vi "科学计算器.vi"() -> ()   [LabVIEW 2014]
panel:
  in  "右":T1
  in  "左":bool
  in  "↓":T2
  in  "↑":bool
  out "结果":string
  out "表达式":string
  in  "OFF":bool
  in  "BACKPLACE":bool
  in  "C":bool
  in  "ln":bool
  in  "^":bool
  in  "tan":bool
  in  "cos":bool
  in  "sin":bool
  in  ")":bool
  in  "(":bool
  in  ".":bool
  in  "=":bool
  in  "0":bool
  in  "9":bool
  in  "8":bool
  in  "7":bool
  in  "6":bool
  in  "5":bool
  in  "4":bool
  in  "3":bool
  in  "2":bool
  in  "1":bool
  in  "÷":bool
  in  "×":bool
  in  "-":bool
  in  "+":bool
  out "数值 2":dbl
  out "数值":dbl
  out "字符串":string
  out "左字":string
  # "小小计算器（科学型）"
  # "ssz"
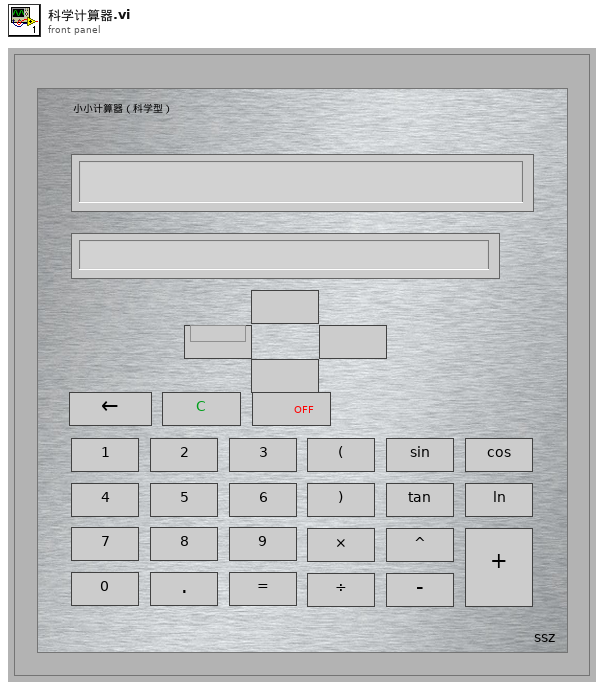
[diagram p1: front panel]
types:
  T1 = typedef "控件 3.ctl" = bool
  T2 = typedef "控件 2.ctl" = bool
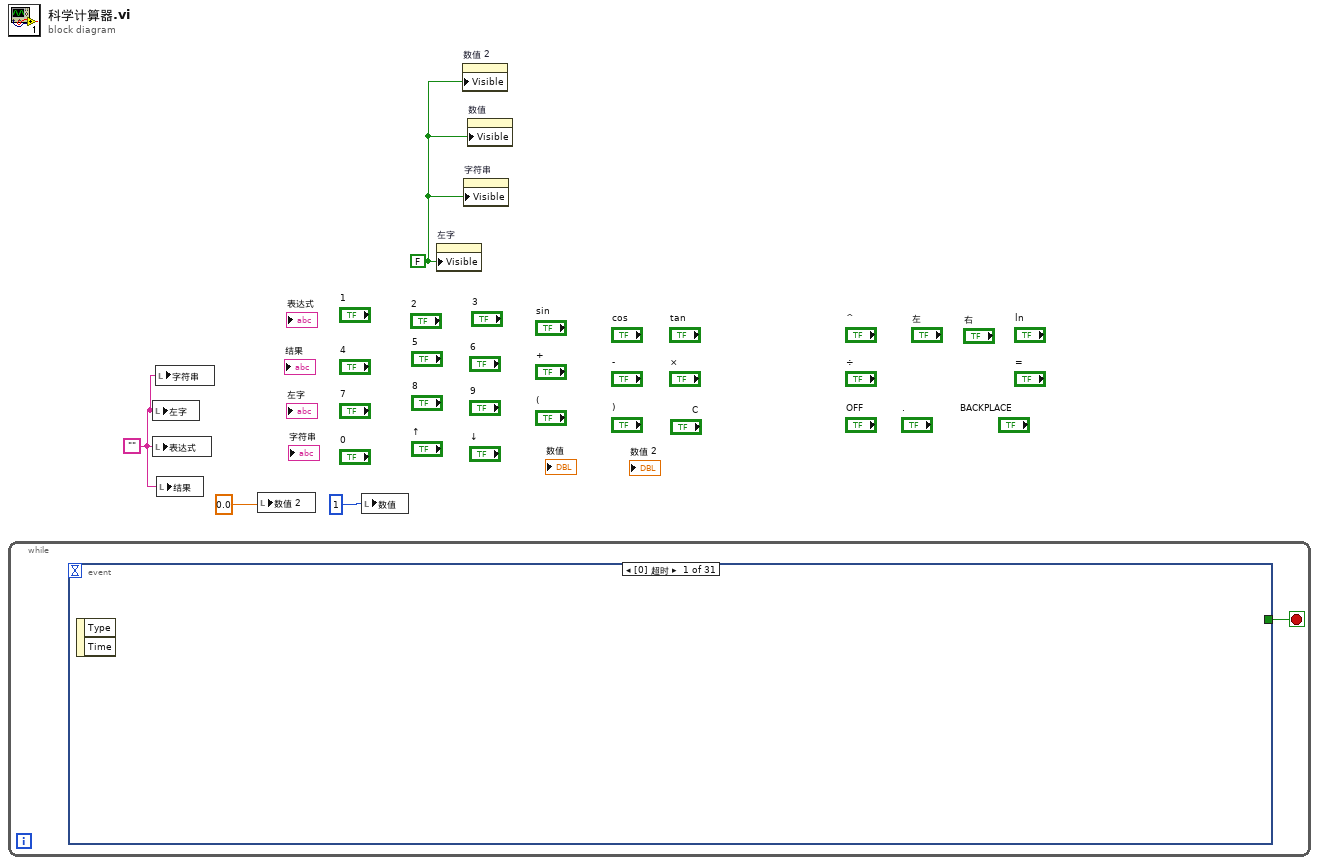
[diagram p0: block diagram]
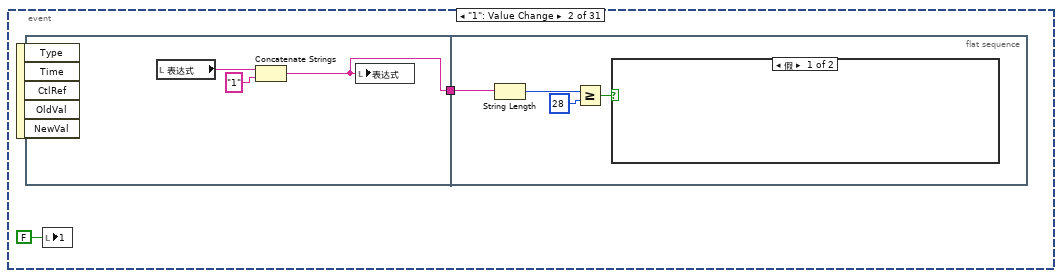
[diagram p2: hidden frame]
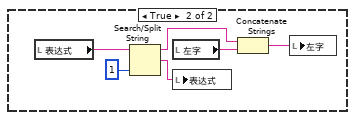
[diagram p3: hidden frame]
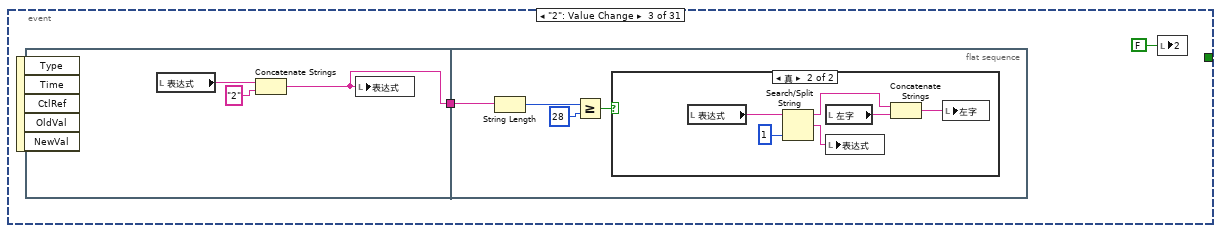
[diagram p4: hidden frame]
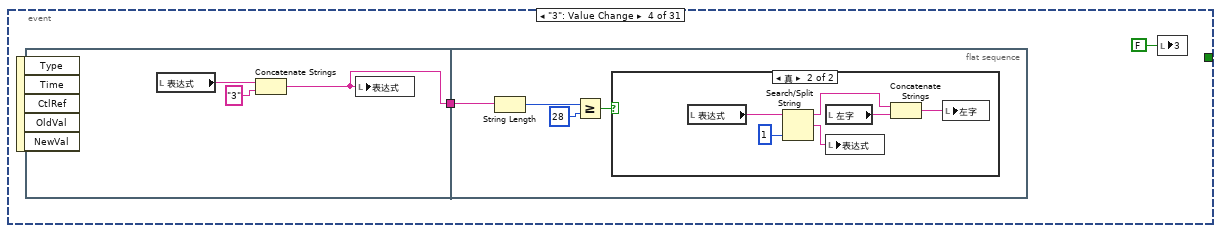
[diagram p6: hidden frame]
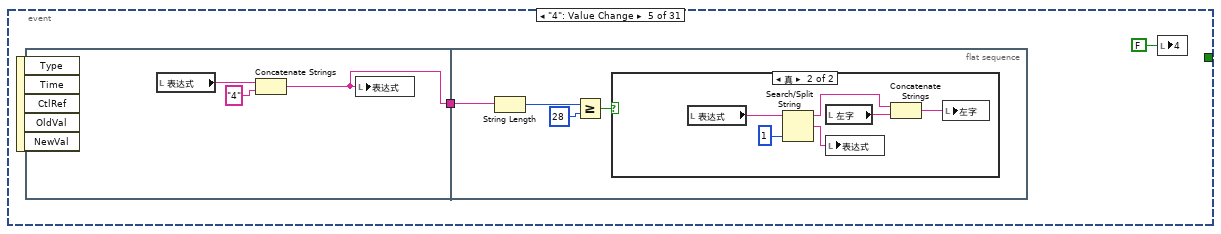
[diagram p8: hidden frame]
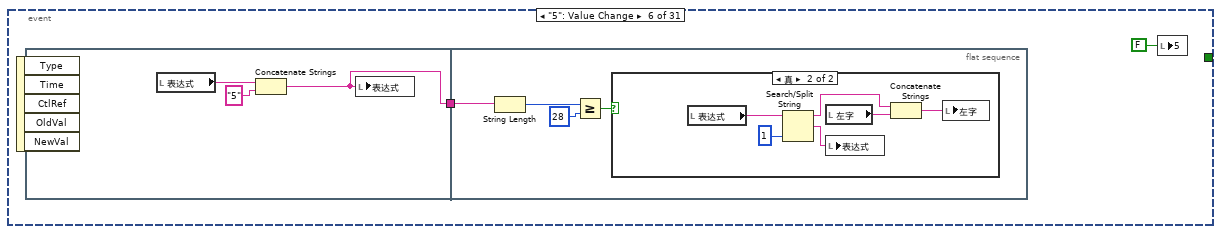
[diagram p10: hidden frame]
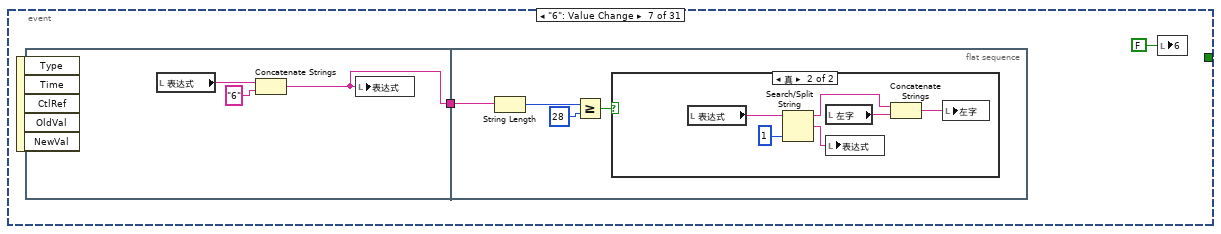
[diagram p12: hidden frame]
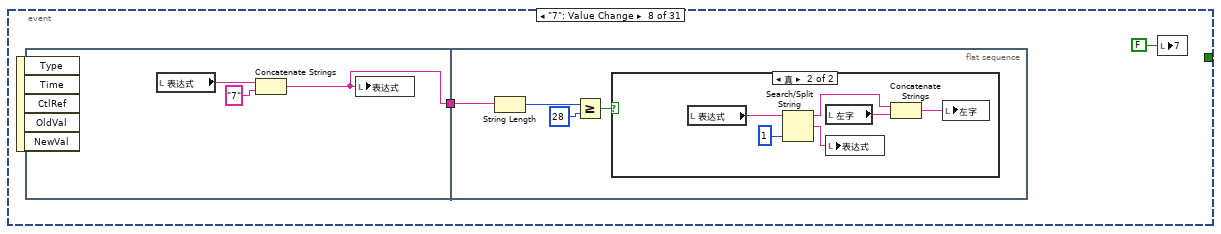
[diagram p14: hidden frame]
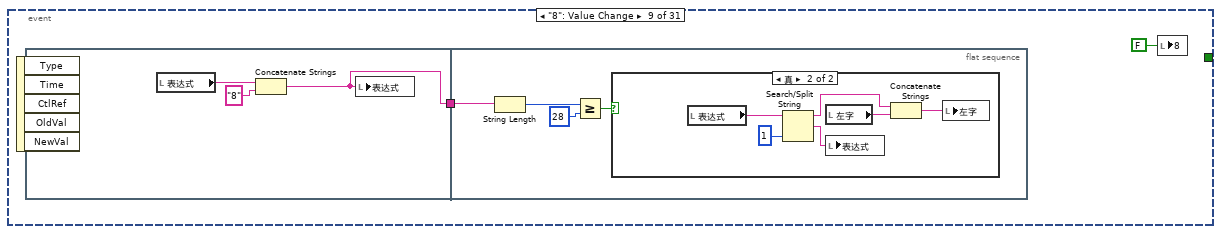
[diagram p16: hidden frame]
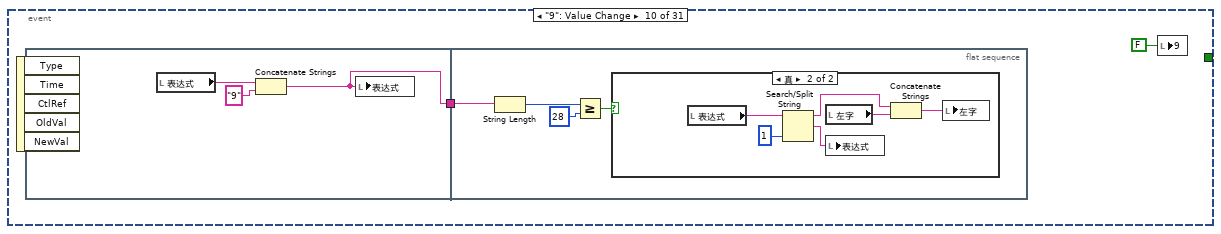
[diagram p18: hidden frame]
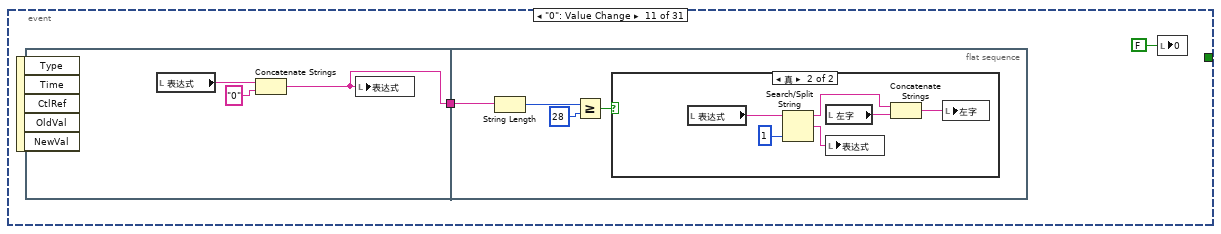
[diagram p20: hidden frame]
diagram:
  w2 = FALSE
  w1 = ""
  n1 = while {
    stop <- w5 stop-if-true
    n2 = event shown="[0] 超时" {
      selector: _ -> [_ _ _ _ _ _ _ _ _ _ _ _ _ _ _ _ _ _ _ _ _ _ _ _ _ _ _ _ _ _ _]
      dyn-events: _ -> [_ _ _ _ _ _ _ _ _ _ _ _ _ _ _ _ _ _ _ _ _ _ _ _ _ _ _ _ _ _ _]
      timeout: _ -> [_ _ _ _ _ _ _ _ _ _ _ _ _ _ _ _ _ _ _ _ _ _ _ _ _ _ _ _ _ _ _]
      tunnel: [_ _ _ _ _ _ _ _ _ _ _ TRUE _ _ _ _ _ _ _ _ _ _ _ _ _ _ _ _ _ _ _] -> w5
      event Timeout {
        n3 = event-data() -> ()  [unwired: 1 in, 2 out]
      }
      event "1": Value Change {
        n4 = event-data() -> ()  [unwired: 1 in, 5 out]
        n5 = flat-sequence {
          tunnel: [w8] -> w6
          tunnel: w6 -> [w11]
          frame #0 {
            n6 = local read "表达式"() -> (w10:string)
            n7 = Concatenate Strings(w10, "1" ("字符串")) -> (w8:string)
            n8 = local write "表达式"(w8) -> ()
          }
          frame #1 {
            n9 = String Length(string=w11) -> (length=w12:i32)
            n10 = Greater Or Equal?(x=w12, y=28) -> (x >= y?=w14:bool)
            n11 = case shown="假" w14 {
              frame False {
              }
              frame True {
                n12 = local read "表达式"() -> (w16:string)
                n13 = Search/Split String(string=w16, offset (0)=1 ("偏移量(0)")) -> (substring before match=w18:string, match + rest of string=w19:string)  [unwired: 1 in, 1 out]
                n14 = local read "左字"() -> (w15:string)
                n15 = local write "表达式"(w19) -> ()
                n16 = Concatenate Strings(w18, w15) -> (w17:string)
                n17 = local write "左字"(w17) -> ()
              }
            }
          }
        }
        n18 = local write "1"(FALSE) -> ()
      }
      event "2": Value Change {
        n19 = event-data() -> ()  [unwired: 1 in, 5 out]
        n20 = flat-sequence {
          tunnel: [w23] -> w21
          tunnel: w21 -> [w26]
          frame #0 {
            n21 = local read "表达式"() -> (w25:string)
            n22 = Concatenate Strings(w25, "2" ("字符串")) -> (w23:string)
            n23 = local write "表达式"(w23) -> ()
          }
          frame #1 {
            n24 = String Length(string=w26) -> (length=w27:i32)
            n25 = Greater Or Equal?(x=w27, y=28) -> (x >= y?=w29:bool)
            n26 = case shown="真" w29 {
              frame False {
              }
              frame True {
                n27 = local read "表达式"() -> (w31:string)
                n28 = Search/Split String(string=w31, offset (0)=1 ("偏移量(0)")) -> (substring before match=w33:string, match + rest of string=w34:string)  [unwired: 1 in, 1 out]
                n29 = local read "左字"() -> (w30:string)
                n30 = local write "表达式"(w34) -> ()
                n31 = Concatenate Strings(w33, w30) -> (w32:string)
                n32 = local write "左字"(w32) -> ()
              }
            }
          }
        }
        n33 = local write "2"(FALSE) -> ()
      }
      event "3": Value Change {
        n34 = event-data() -> ()  [unwired: 1 in, 5 out]
        n35 = flat-sequence {
          tunnel: [w38] -> w36
          tunnel: w36 -> [w41]
          frame #0 {
            n36 = local read "表达式"() -> (w40:string)
            n37 = Concatenate Strings(w40, "3" ("字符串")) -> (w38:string)
            n38 = local write "表达式"(w38) -> ()
          }
          frame #1 {
            n39 = String Length(string=w41) -> (length=w42:i32)
            n40 = Greater Or Equal?(x=w42, y=28) -> (x >= y?=w44:bool)
            n41 = case shown="真" w44 {
              frame False {
              }
              frame True {
                n42 = local read "表达式"() -> (w46:string)
                n43 = Search/Split String(string=w46, offset (0)=1 ("偏移量(0)")) -> (substring before match=w48:string, match + rest of string=w49:string)  [unwired: 1 in, 1 out]
                n44 = local read "左字"() -> (w45:string)
                n45 = local write "表达式"(w49) -> ()
                n46 = Concatenate Strings(w48, w45) -> (w47:string)
                n47 = local write "左字"(w47) -> ()
              }
            }
          }
        }
        n48 = local write "3"(FALSE) -> ()
      }
      event "4": Value Change {
        n49 = event-data() -> ()  [unwired: 1 in, 5 out]
        n50 = flat-sequence {
          tunnel: [w53] -> w51
          tunnel: w51 -> [w56]
          frame #0 {
            n51 = local read "表达式"() -> (w55:string)
            n52 = Concatenate Strings(w55, "4" ("字符串")) -> (w53:string)
            n53 = local write "表达式"(w53) -> ()
          }
          frame #1 {
            n54 = String Length(string=w56) -> (length=w57:i32)
            n55 = Greater Or Equal?(x=w57, y=28) -> (x >= y?=w59:bool)
            n56 = case shown="真" w59 {
              frame False {
              }
              frame True {
                n57 = local read "表达式"() -> (w61:string)
                n58 = Search/Split String(string=w61, offset (0)=1 ("偏移量(0)")) -> (substring before match=w63:string, match + rest of string=w64:string)  [unwired: 1 in, 1 out]
                n59 = local read "左字"() -> (w60:string)
                n60 = local write "表达式"(w64) -> ()
                n61 = Concatenate Strings(w63, w60) -> (w62:string)
                n62 = local write "左字"(w62) -> ()
              }
            }
          }
        }
        n63 = local write "4"(FALSE ("4")) -> ()
      }
      event "5": Value Change {
        n64 = event-data() -> ()  [unwired: 1 in, 5 out]
        n65 = flat-sequence {
          tunnel: [w68] -> w66
          tunnel: w66 -> [w71]
          frame #0 {
            n66 = local read "表达式"() -> (w70:string)
            n67 = Concatenate Strings(w70, "5" ("字符串")) -> (w68:string)
            n68 = local write "表达式"(w68) -> ()
          }
          frame #1 {
            n69 = String Length(string=w71) -> (length=w72:i32)
            n70 = Greater Or Equal?(x=w72, y=28) -> (x >= y?=w74:bool)
            n71 = case shown="真" w74 {
              frame False {
              }
              frame True {
                n72 = local read "表达式"() -> (w76:string)
                n73 = Search/Split String(string=w76, offset (0)=1 ("偏移量(0)")) -> (substring before match=w78:string, match + rest of string=w79:string)  [unwired: 1 in, 1 out]
                n74 = local read "左字"() -> (w75:string)
                n75 = local write "表达式"(w79) -> ()
                n76 = Concatenate Strings(w78, w75) -> (w77:string)
                n77 = local write "左字"(w77) -> ()
              }
            }
          }
        }
        n78 = local write "5"(FALSE ("5")) -> ()
      }
      event "6": Value Change {
        n79 = event-data() -> ()  [unwired: 1 in, 5 out]
        n80 = flat-sequence {
          tunnel: [w83] -> w81
          tunnel: w81 -> [w86]
          frame #0 {
            n81 = local read "表达式"() -> (w85:string)
            n82 = Concatenate Strings(w85, "6" ("字符串")) -> (w83:string)
            n83 = local write "表达式"(w83) -> ()
          }
          frame #1 {
            n84 = String Length(string=w86) -> (length=w87:i32)
            n85 = Greater Or Equal?(x=w87, y=28) -> (x >= y?=w89:bool)
            n86 = case shown="真" w89 {
              frame False {
              }
              frame True {
                n87 = local read "表达式"() -> (w91:string)
                n88 = Search/Split String(string=w91, offset (0)=1 ("偏移量(0)")) -> (substring before match=w93:string, match + rest of string=w94:string)  [unwired: 1 in, 1 out]
                n89 = local read "左字"() -> (w90:string)
                n90 = local write "表达式"(w94) -> ()
                n91 = Concatenate Strings(w93, w90) -> (w92:string)
                n92 = local write "左字"(w92) -> ()
              }
            }
          }
        }
        n93 = local write "6"(FALSE ("6")) -> ()
      }
      event "7": Value Change {
        n94 = event-data() -> ()  [unwired: 1 in, 5 out]
        n95 = flat-sequence {
          tunnel: [w98] -> w96
          tunnel: w96 -> [w101]
          frame #0 {
            n96 = local read "表达式"() -> (w100:string)
            n97 = Concatenate Strings(w100, "7" ("字符串")) -> (w98:string)
            n98 = local write "表达式"(w98) -> ()
          }
          frame #1 {
            n99 = String Length(string=w101) -> (length=w102:i32)
            n100 = Greater Or Equal?(x=w102, y=28) -> (x >= y?=w104:bool)
            n101 = case shown="真" w104 {
              frame False {
              }
              frame True {
                n102 = local read "表达式"() -> (w106:string)
                n103 = Search/Split String(string=w106, offset (0)=1 ("偏移量(0)")) -> (substring before match=w108:string, match + rest of string=w109:string)  [unwired: 1 in, 1 out]
                n104 = local read "左字"() -> (w105:string)
                n105 = local write "表达式"(w109) -> ()
                n106 = Concatenate Strings(w108, w105) -> (w107:string)
                n107 = local write "左字"(w107) -> ()
              }
            }
          }
        }
        n108 = local write "7"(FALSE ("7")) -> ()
      }
      event "8": Value Change {
        n109 = event-data() -> ()  [unwired: 1 in, 5 out]
        n110 = flat-sequence {
          tunnel: [w113] -> w111
          tunnel: w111 -> [w116]
          frame #0 {
            n111 = local read "表达式"() -> (w115:string)
            n112 = Concatenate Strings(w115, "8" ("字符串")) -> (w113:string)
            n113 = local write "表达式"(w113) -> ()
          }
          frame #1 {
            n114 = String Length(string=w116) -> (length=w117:i32)
            n115 = Greater Or Equal?(x=w117, y=28) -> (x >= y?=w119:bool)
            n116 = case shown="真" w119 {
              frame False {
              }
              frame True {
                n117 = local read "表达式"() -> (w121:string)
                n118 = Search/Split String(string=w121, offset (0)=1 ("偏移量(0)")) -> (substring before match=w123:string, match + rest of string=w124:string)  [unwired: 1 in, 1 out]
                n119 = local read "左字"() -> (w120:string)
                n120 = local write "表达式"(w124) -> ()
                n121 = Concatenate Strings(w123, w120) -> (w122:string)
                n122 = local write "左字"(w122) -> ()
              }
            }
          }
        }
        n123 = local write "8"(FALSE ("8")) -> ()
      }
      event "9": Value Change {
        n124 = event-data() -> ()  [unwired: 1 in, 5 out]
        n125 = flat-sequence {
          tunnel: [w128] -> w126
          tunnel: w126 -> [w131]
          frame #0 {
            n126 = local read "表达式"() -> (w130:string)
            n127 = Concatenate Strings(w130, "9" ("字符串")) -> (w128:string)
            n128 = local write "表达式"(w128) -> ()
          }
          frame #1 {
            n129 = String Length(string=w131) -> (length=w132:i32)
            n130 = Greater Or Equal?(x=w132, y=28) -> (x >= y?=w134:bool)
            n131 = case shown="真" w134 {
              frame False {
              }
              frame True {
                n132 = local read "表达式"() -> (w136:string)
                n133 = Search/Split String(string=w136, offset (0)=1 ("偏移量(0)")) -> (substring before match=w138:string, match + rest of string=w139:string)  [unwired: 1 in, 1 out]
                n134 = local read "左字"() -> (w135:string)
                n135 = local write "表达式"(w139) -> ()
                n136 = Concatenate Strings(w138, w135) -> (w137:string)
                n137 = local write "左字"(w137) -> ()
              }
            }
          }
        }
        n138 = local write "9"(FALSE ("9")) -> ()
      }
      event "0": Value Change {
        n139 = event-data() -> ()  [unwired: 1 in, 5 out]
        n140 = flat-sequence {
          tunnel: [w143] -> w141
          tunnel: w141 -> [w146]
          frame #0 {
            n141 = local read "表达式"() -> (w145:string)
            n142 = Concatenate Strings(w145, "0" ("字符串")) -> (w143:string)
            n143 = local write "表达式"(w143) -> ()
          }
          frame #1 {
            n144 = String Length(string=w146) -> (length=w147:i32)
            n145 = Greater Or Equal?(x=w147, y=28) -> (x >= y?=w149:bool)
            n146 = case shown="真" w149 {
              frame False {
              }
              frame True {
                n147 = local read "表达式"() -> (w151:string)
                n148 = Search/Split String(string=w151, offset (0)=1 ("偏移量(0)")) -> (substring before match=w153:string, match + rest of string=w154:string)  [unwired: 1 in, 1 out]
                n149 = local read "左字"() -> (w150:string)
                n150 = local write "表达式"(w154) -> ()
                n151 = Concatenate Strings(w153, w150) -> (w152:string)
                n152 = local write "左字"(w152) -> ()
              }
            }
          }
        }
        n153 = local write "0"(FALSE ("0")) -> ()
      }
      event "OFF": Value Change {
        n154 = event-data() -> ()  [unwired: 1 in, 5 out]
        n155 = local write "OFF"(FALSE ("OFF")) -> ()
      }
      event "sin": Value Change {
        n156 = event-data() -> ()  [unwired: 1 in, 5 out]
        n157 = flat-sequence {
          tunnel: [w160] -> w158
          tunnel: w158 -> [w163]
          frame #0 {
            n158 = local read "表达式"() -> (w162:string)
            n159 = Concatenate Strings(w162, "sin" ("字符串")) -> (w160:string)
            n160 = local write "表达式"(w160) -> ()
          }
          frame #1 {
            n161 = String Length(string=w163) -> (length=w164:i32)
            n162 = Greater Or Equal?(x=w164, y=28) -> (x >= y?=w166:bool)
            n163 = case shown="真" w166 {
              frame False {
              }
              frame True {
                n164 = local read "表达式"() -> (w168:string)
                n165 = Search/Split String(string=w168, offset (0)=1 ("偏移量(0)")) -> (substring before match=w170:string, match + rest of string=w171:string)  [unwired: 1 in, 1 out]
                n166 = local read "左字"() -> (w167:string)
                n167 = local write "表达式"(w171) -> ()
                n168 = Concatenate Strings(w170, w167) -> (w169:string)
                n169 = local write "左字"(w169) -> ()
              }
            }
          }
        }
        n170 = local write "sin"(FALSE) -> ()
      }
      event "↑": Value Change {
        n171 = event-data() -> ()  [unwired: 1 in, 5 out]
        n172 = flat-sequence {
          frame #0 {
            n173 = local read "数值"() -> (w175:dbl)
            n174 = local read "字符串"() -> (w177:string)
            n175 = Increment(x=w175) -> (x+1=w174:dbl)
            n176 = Pick Line(multi-line string=w177, line index=w175) -> (output string=w176:string)  [unwired: 1 in]
            n177 = local write "数值"(w174) -> ()
            n178 = local write "表达式"(w176) -> ()
          }
          frame #1 {
            n179 = local read "数值"() -> (w180:dbl)
            n180 = Subtract(x=w180, y=2) -> (x-y=w179:dbl)
            n181 = local write "数值 2"(w179) -> ()
          }
        }
        n182 = local write "↑"(FALSE) -> ()
      }
      event "cos": Value Change {
        n183 = event-data() -> ()  [unwired: 1 in, 5 out]
        n184 = flat-sequence {
          tunnel: [w183] -> w181
          tunnel: w181 -> [w186]
          frame #0 {
            n185 = local read "表达式"() -> (w185:string)
            n186 = Concatenate Strings(w185, "cos" ("字符串")) -> (w183:string)
            n187 = local write "表达式"(w183) -> ()
          }
          frame #1 {
            n188 = String Length(string=w186) -> (length=w187:i32)
            n189 = Greater Or Equal?(x=w187, y=28) -> (x >= y?=w189:bool)
            n190 = case shown="真" w189 {
              frame False {
              }
              frame True {
                n191 = local read "表达式"() -> (w191:string)
                n192 = Search/Split String(string=w191, offset (0)=1 ("偏移量(0)")) -> (substring before match=w193:string, match + rest of string=w194:string)  [unwired: 1 in, 1 out]
                n193 = local read "左字"() -> (w190:string)
                n194 = local write "表达式"(w194) -> ()
                n195 = Concatenate Strings(w193, w190) -> (w192:string)
                n196 = local write "左字"(w192) -> ()
              }
            }
          }
        }
        n197 = local write "cos"(FALSE ("cos")) -> ()
      }
      event "tan": Value Change {
        n198 = event-data() -> ()  [unwired: 1 in, 5 out]
        n199 = flat-sequence {
          tunnel: [w198] -> w196
          tunnel: w196 -> [w201]
          frame #0 {
            n200 = local read "表达式"() -> (w200:string)
            n201 = Concatenate Strings(w200, "tan" ("字符串")) -> (w198:string)
            n202 = local write "表达式"(w198) -> ()
          }
          frame #1 {
            n203 = String Length(string=w201) -> (length=w202:i32)
            n204 = Greater Or Equal?(x=w202, y=28) -> (x >= y?=w204:bool)
            n205 = case shown="真" w204 {
              frame False {
              }
              frame True {
                n206 = local read "表达式"() -> (w206:string)
                n207 = Search/Split String(string=w206, offset (0)=1 ("偏移量(0)")) -> (substring before match=w208:string, match + rest of string=w209:string)  [unwired: 1 in, 1 out]
                n208 = local read "左字"() -> (w205:string)
                n209 = local write "表达式"(w209) -> ()
                n210 = Concatenate Strings(w208, w205) -> (w207:string)
                n211 = local write "左字"(w207) -> ()
              }
            }
          }
        }
        n212 = local write "tan"(FALSE ("tan")) -> ()
      }
      event "^": Value Change {
        n213 = event-data() -> ()  [unwired: 1 in, 5 out]
        n214 = flat-sequence {
          tunnel: [w213] -> w211
          tunnel: w211 -> [w216]
          frame #0 {
            n215 = local read "表达式"() -> (w215:string)
            n216 = Concatenate Strings(w215, "^" ("字符串")) -> (w213:string)
            n217 = local write "表达式"(w213) -> ()
          }
          frame #1 {
            n218 = String Length(string=w216) -> (length=w217:i32)
            n219 = Greater Or Equal?(x=w217, y=28) -> (x >= y?=w219:bool)
            n220 = case shown="真" w219 {
              frame False {
              }
              frame True {
                n221 = local read "表达式"() -> (w221:string)
                n222 = Search/Split String(string=w221, offset (0)=1 ("偏移量(0)")) -> (substring before match=w223:string, match + rest of string=w224:string)  [unwired: 1 in, 1 out]
                n223 = local read "左字"() -> (w220:string)
                n224 = local write "表达式"(w224) -> ()
                n225 = Concatenate Strings(w223, w220) -> (w222:string)
                n226 = local write "左字"(w222) -> ()
              }
            }
          }
        }
        n227 = local write "^"(FALSE ("e^x")) -> ()
      }
      event "ln": Value Change {
        n228 = event-data() -> ()  [unwired: 1 in, 5 out]
        n229 = flat-sequence {
          tunnel: [w228] -> w226
          tunnel: w226 -> [w231]
          frame #0 {
            n230 = local read "表达式"() -> (w230:string)
            n231 = Concatenate Strings(w230, "ln" ("字符串")) -> (w228:string)
            n232 = local write "表达式"(w228) -> ()
          }
          frame #1 {
            n233 = String Length(string=w231) -> (length=w232:i32)
            n234 = Greater Or Equal?(x=w232, y=28) -> (x >= y?=w234:bool)
            n235 = case shown="真" w234 {
              frame False {
              }
              frame True {
                n236 = local read "表达式"() -> (w236:string)
                n237 = Search/Split String(string=w236, offset (0)=1 ("偏移量(0)")) -> (substring before match=w238:string, match + rest of string=w239:string)  [unwired: 1 in, 1 out]
                n238 = local read "左字"() -> (w235:string)
                n239 = local write "表达式"(w239) -> ()
                n240 = Concatenate Strings(w238, w235) -> (w237:string)
                n241 = local write "左字"(w237) -> ()
              }
            }
          }
        }
        n242 = local write "ln"(FALSE ("ln")) -> ()
      }
      event "左": Value Change {
        n243 = event-data() -> ()  [unwired: 1 in, 2 out]
        n244 = local read "表达式"() -> (w243:string)
        n245 = Search/Split String(string=w243, offset (0)=1 ("偏移量(0)")) -> (substring before match=w245:string, match + rest of string=w246:string)  [unwired: 1 in, 1 out]
        n246 = local write "表达式"(w246) -> ()
        n247 = local read "左字"() -> (w242:string)
        n248 = Concatenate Strings(w245, w242) -> (w244:string)
        n249 = local write "左字"(w244) -> ()
        n250 = local write "左"(FALSE) -> ()
      }
      event Value Change {
        n251 = event-data() -> ()  [unwired: 1 in, 5 out]
        n252 = local read "左字"() -> (w256:string)
        n253 = local read "表达式"() -> (w252:string)
        n254 = Search/Split String(string=w256, offset (0)=1 ("偏移量(0)")) -> (substring before match=w254:string, match + rest of string=w253:string)  [unwired: 1 in, 1 out]
        n255 = local write "左字"(w253) -> ()
        n256 = Reverse String(1:w252) -> (0:w251:string)
        n257 = Concatenate Strings(w251, w254) -> (w250:string)
        n258 = Reverse String(1:w250) -> (0:w249:string)
        n259 = local write "表达式"(w249) -> ()
        n260 = local write "右"(FALSE) -> ()
      }
      event "C": Value Change {
        w257 = ""
        n261 = event-data() -> ()  [unwired: 1 in, 5 out]
        n262 = local write "左字"(w257) -> ()
        n263 = local write "结果"(w257) -> ()
        n264 = local write "表达式"(w257) -> ()
        n265 = local write "C"(FALSE) -> ()
      }
      event ".": Value Change {
        n266 = event-data() -> ()  [unwired: 1 in, 5 out]
        n267 = flat-sequence {
          tunnel: [w261] -> w259
          tunnel: w259 -> [w264]
          frame #0 {
            n268 = local read "表达式"() -> (w263:string)
            n269 = Concatenate Strings(w263, "." ("字符串")) -> (w261:string)
            n270 = local write "表达式"(w261) -> ()
          }
          frame #1 {
            n271 = String Length(string=w264) -> (length=w265:i32)
            n272 = Greater Or Equal?(x=w265, y=28) -> (x >= y?=w267:bool)
            n273 = case shown="真" w267 {
              frame False {
              }
              frame True {
                n274 = local read "表达式"() -> (w269:string)
                n275 = Search/Split String(string=w269, offset (0)=1 ("偏移量(0)")) -> (substring before match=w271:string, match + rest of string=w272:string)  [unwired: 1 in, 1 out]
                n276 = local write "表达式"(w272) -> ()
                n277 = local read "左字"() -> (w268:string)
                n278 = Concatenate Strings(w271, w268) -> (w270:string)
                n279 = local write "左字"(w270) -> ()
              }
            }
          }
        }
        n280 = local write "."(FALSE (".")) -> ()
      }
      event "(": Value Change {
        n281 = event-data() -> ()  [unwired: 1 in, 5 out]
        n282 = flat-sequence {
          tunnel: [w276] -> w274
          tunnel: w274 -> [w279]
          frame #0 {
            n283 = local read "表达式"() -> (w278:string)
            n284 = Concatenate Strings(w278, "(" ("字符串")) -> (w276:string)
            n285 = local write "表达式"(w276) -> ()
          }
          frame #1 {
            n286 = String Length(string=w279) -> (length=w280:i32)
            n287 = Greater Or Equal?(x=w280, y=28) -> (x >= y?=w282:bool)
            n288 = case shown="真" w282 {
              frame False {
              }
              frame True {
                n289 = local read "表达式"() -> (w284:string)
                n290 = Search/Split String(string=w284, offset (0)=1 ("偏移量(0)")) -> (substring before match=w286:string, match + rest of string=w287:string)  [unwired: 1 in, 1 out]
                n291 = local write "表达式"(w287) -> ()
                n292 = local read "左字"() -> (w283:string)
                n293 = Concatenate Strings(w286, w283) -> (w285:string)
                n294 = local write "左字"(w285) -> ()
              }
            }
          }
        }
        n295 = local write "("(FALSE ("(")) -> ()
      }
      event ")": Value Change {
        n296 = event-data() -> ()  [unwired: 1 in, 5 out]
        n297 = flat-sequence {
          tunnel: [w291] -> w289
          tunnel: w289 -> [w294]
          frame #0 {
            n298 = local read "表达式"() -> (w293:string)
            n299 = Concatenate Strings(w293, ")" ("字符串")) -> (w291:string)
            n300 = local write "表达式"(w291) -> ()
          }
          frame #1 {
            n301 = String Length(string=w294) -> (length=w295:i32)
            n302 = Greater Or Equal?(x=w295, y=28) -> (x >= y?=w297:bool)
            n303 = case shown="真" w297 {
              frame False {
              }
              frame True {
                n304 = local read "表达式"() -> (w299:string)
                n305 = Search/Split String(string=w299, offset (0)=1 ("偏移量(0)")) -> (substring before match=w301:string, match + rest of string=w302:string)  [unwired: 1 in, 1 out]
                n306 = local write "表达式"(w302) -> ()
                n307 = local read "左字"() -> (w298:string)
                n308 = Concatenate Strings(w301, w298) -> (w300:string)
                n309 = local write "左字"(w300) -> ()
              }
            }
          }
        }
        n310 = local write ")"(FALSE (")")) -> ()
      }
      event "+": Value Change {
        n311 = event-data() -> ()  [unwired: 1 in, 5 out]
        n312 = flat-sequence {
          tunnel: [w306] -> w304
          tunnel: w304 -> [w309]
          frame #0 {
            n313 = local read "表达式"() -> (w308:string)
            n314 = Concatenate Strings(w308, "+" ("字符串")) -> (w306:string)
            n315 = local write "表达式"(w306) -> ()
          }
          frame #1 {
            n316 = String Length(string=w309) -> (length=w310:i32)
            n317 = Greater Or Equal?(x=w310, y=28) -> (x >= y?=w312:bool)
            n318 = case shown="真" w312 {
              frame False {
              }
              frame True {
                n319 = local read "表达式"() -> (w314:string)
                n320 = Search/Split String(string=w314, offset (0)=1 ("偏移量(0)")) -> (substring before match=w316:string, match + rest of string=w317:string)  [unwired: 1 in, 1 out]
                n321 = local read "左字"() -> (w313:string)
                n322 = local write "表达式"(w317) -> ()
                n323 = Concatenate Strings(w316, w313) -> (w315:string)
                n324 = local write "左字"(w315) -> ()
              }
            }
          }
        }
        n325 = local write "+"(FALSE ("+")) -> ()
      }
      event "-": Value Change {
        n326 = event-data() -> ()  [unwired: 1 in, 5 out]
        n327 = flat-sequence {
          tunnel: [w321] -> w319
          tunnel: w319 -> [w324]
          frame #0 {
            n328 = local read "表达式"() -> (w323:string)
            n329 = Concatenate Strings(w323, "-" ("字符串")) -> (w321:string)
            n330 = local write "表达式"(w321) -> ()
          }
          frame #1 {
            n331 = String Length(string=w324) -> (length=w325:i32)
            n332 = Greater Or Equal?(x=w325, y=28) -> (x >= y?=w327:bool)
            n333 = case shown="真" w327 {
              frame False {
              }
              frame True {
                n334 = local read "表达式"() -> (w329:string)
                n335 = Search/Split String(string=w329, offset (0)=1 ("偏移量(0)")) -> (substring before match=w331:string, match + rest of string=w332:string)  [unwired: 1 in, 1 out]
                n336 = local write "表达式"(w332) -> ()
                n337 = local read "左字"() -> (w328:string)
                n338 = Concatenate Strings(w331, w328) -> (w330:string)
                n339 = local write "左字"(w330) -> ()
              }
            }
          }
        }
        n340 = local write "-"(FALSE ("-")) -> ()
      }
      event "×": Value Change {
        n341 = event-data() -> ()  [unwired: 1 in, 5 out]
        n342 = flat-sequence {
          tunnel: [w336] -> w334
          tunnel: w334 -> [w339]
          frame #0 {
            n343 = local read "表达式"() -> (w338:string)
            n344 = Concatenate Strings(w338, "*" ("字符串")) -> (w336:string)
            n345 = local write "表达式"(w336) -> ()
          }
          frame #1 {
            n346 = String Length(string=w339) -> (length=w340:i32)
            n347 = Greater Or Equal?(x=w340, y=28) -> (x >= y?=w342:bool)
            n348 = case shown="真" w342 {
              frame False {
              }
              frame True {
                n349 = local read "表达式"() -> (w344:string)
                n350 = Search/Split String(string=w344, offset (0)=1 ("偏移量(0)")) -> (substring before match=w346:string, match + rest of string=w347:string)  [unwired: 1 in, 1 out]
                n351 = local write "表达式"(w347) -> ()
                n352 = local read "左字"() -> (w343:string)
                n353 = Concatenate Strings(w346, w343) -> (w345:string)
                n354 = local write "左字"(w345) -> ()
              }
            }
          }
        }
        n355 = local write "×"(FALSE ("×")) -> ()
      }
      event "÷": Value Change {
        n356 = event-data() -> ()  [unwired: 1 in, 5 out]
        n357 = flat-sequence {
          tunnel: [w351] -> w349
          tunnel: w349 -> [w354]
          frame #0 {
            n358 = local read "表达式"() -> (w353:string)
            n359 = Concatenate Strings(w353, "/" ("字符串")) -> (w351:string)
            n360 = local write "表达式"(w351) -> ()
          }
          frame #1 {
            n361 = String Length(string=w354) -> (length=w355:i32)
            n362 = Greater Or Equal?(x=w355, y=28) -> (x >= y?=w357:bool)
            n363 = case shown="真" w357 {
              frame False {
              }
              frame True {
                n364 = local read "表达式"() -> (w359:string)
                n365 = Search/Split String(string=w359, offset (0)=1 ("偏移量(0)")) -> (substring before match=w361:string, match + rest of string=w362:string)  [unwired: 1 in, 1 out]
                n366 = local write "表达式"(w362) -> ()
                n367 = local read "左字"() -> (w358:string)
                n368 = Concatenate Strings(w361, w358) -> (w360:string)
                n369 = local write "左字"(w360) -> ()
              }
            }
          }
        }
        n370 = local write "÷"(FALSE ("÷")) -> ()
      }
      event "=": Value Change {
        n371 = event-data() -> ()  [unwired: 1 in, 5 out]
        n372 = local read "左字"() -> (w372:string)
        n373 = local read "表达式"() -> (w370:string)
        n374 = Reverse String(1:w372) -> (0:w371:string)
        n375 = local read "字符串"() -> (w365:string)
        n376 = Concatenate Strings(w371, w370) -> (w366:string)
        n377 = call "括号.vi"("表达式"=w366) -> ("结果"=w368:string)
        n378 = local write "结果"(w368) -> ()
        n379 = Concatenate Strings("\r\n", w366, w365) -> (w367:string)
        n380 = local write "字符串"(w367) -> ()
        n381 = local write "="(FALSE) -> ()
      }
      event Value Change {
        n382 = event-data() -> ()  [unwired: 1 in, 5 out]
        n383 = flat-sequence {
          frame #0 {
            n384 = local read "数值 2"() -> (w375:dbl)
            n385 = local read "字符串"() -> (w377:string)
            n386 = Decrement(x=w375) -> (x-1=w374:dbl)
            n387 = Pick Line(multi-line string=w377, line index=w375) -> (output string=w376:string)  [unwired: 1 in]
            n388 = local write "数值 2"(w374) -> ()
            n389 = local write "表达式"(w376) -> ()
          }
          frame #1 {
            n390 = local read "数值 2"() -> (w379:dbl)
            n391 = Add(x=w379, y=2.0) -> (x+y=w380:dbl)
            n392 = local write "数值"(w380) -> ()
          }
        }
        n393 = local write "↓"(FALSE) -> ()
      }
      event "BACKPLACE": Value Change {
        n394 = event-data() -> ()  [unwired: 1 in, 5 out]
        n395 = local write "BACKPLACE"(FALSE ("BACKPLACE")) -> ()
        n396 = local read "表达式"() -> (w385:string)
        n397 = String Length(string=w385) -> (length=w384:i32)
        n398 = Subtract(x=w384, y=1 ("长度（剩余）")) -> (x-y=w382:i32)
        n399 = String Subset(string=w385, length (rest)=w382) -> (substring=w386:string)  [unwired: 1 in]
        n400 = local write "表达式"(w386) -> ()
      }
    }
  }
  n401 = local write "左字"(w1) -> ()
  n402 = local write "表达式"(w1) -> ()
  n403 = local write "字符串"(w1) -> ()
  n404 = local write "结果"(w1) -> ()
  n405 = local write "数值 2"(0.0) -> ()
  n406 = local write "数值"(1) -> ()
  n407 = property on="左字" class="Str"("Visible"=w2) -> ()  [unwired: 2 in, 2 out]
  n408 = property on="数值 2" class="DigNum (严格)"("Visible"=w2) -> ()  [unwired: 2 in, 2 out]
  n409 = property on="字符串" class="Str"("Visible"=w2) -> ()  [unwired: 2 in, 2 out]
  n410 = property on="数值" class="DigNum (严格)"("Visible"=w2) -> ()  [unwired: 2 in, 2 out]
